vi "Add Noise Single.vi"(6 "Sampling":T2 {"Fs" format="%#_13g"}, 8 "error in (no error)":errorcluster, 10 "Noise Cluster":T1={"1/f vs. Uniform "=0.005, "60Hz Amplitude"=0.005, "Gauss/Unif %"=0.5, "Noise Amp"=0.005}, 11 "signal in":waveform(dbl)) -> (0 "error out":errorcluster, 3 "signal out":waveform(dbl))   [LabVIEW 2019, in "DAQmx.lvclass"]
uses:
  DAQmx.lvclass
  Instrument.DAQ/Typedefs/DAQ.Sampling.Sampling--Cluster.ctl
  <vilib>/measure/NI_MABase.lvlib
  Instrument.DAQ/Instrument.DAQ.lvclass
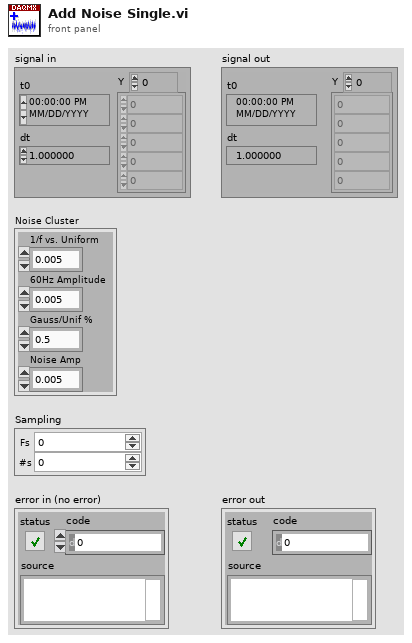
[diagram p1: front panel]
types:
  T1 = cluster{"1/f vs. Uniform ":dbl, "60Hz Amplitude":dbl, "Gauss/Unif %":dbl, "Noise Amp":dbl}
  T2 = typedef "Instrument.Lockin.lvlib/Instrument.DAQ.lvclass/DAQ.Sampling.Sampling--Cluster.ctl" = cluster{"Fs":dbl, "#s":i32}
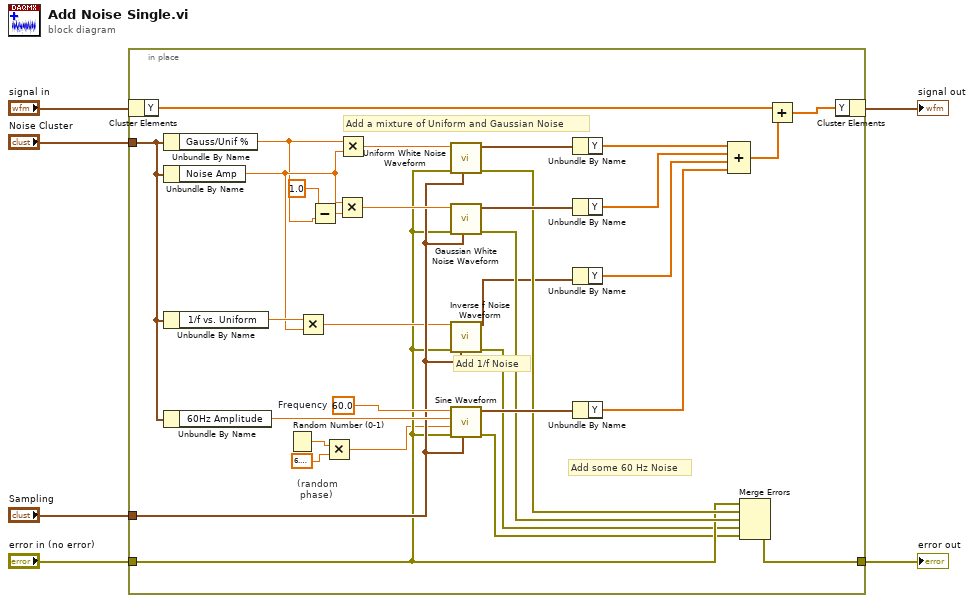
[diagram p0: block diagram]
diagram:
  n1 = in-place {
    in-place-border: "Noise Cluster" -> [w38]
    in-place-border: "Sampling" -> [w21]
    in-place-border: "error in (no error)" -> [w17]
    in-place-border: [w16] -> w4
    w25 = 60.0  # Frequency
    # "(random\n phase)"
    # "Add 1/f Noise"
    # "Add some 60 Hz Noise"
    # "Add a mixture of Uniform and Gaussian Noise"
    n2 = in-place-cluster #1("signal in") -> ("Y"=w14:dbl[])
    n3 = Unbundle By Name(w38) -> ("Gauss/Unif %"=w7:dbl)
    n4 = Unbundle By Name(w38) -> ("Noise Amp"=w22:dbl)
    n5 = Unbundle By Name(w38) -> ("1/f vs. Uniform"=w29:dbl)
    n6 = Unbundle By Name(w38) -> ("60Hz Amplitude"=w28:dbl)
    n7 = Random Number (0-1)() -> (number: 0 to 1=w11:dbl)
    n8 = Multiply(x=w29, y=w22) -> (x*y=w20:dbl)
    n9 = Subtract(x=1.0, y=w7) -> (x-y=w35:dbl)
    n10 = Multiply(x=w11, y=6.283185307179586) -> (x*y=w9:dbl)
    n11 = Multiply(x=w22, y=w35) -> (x*y=w27:dbl)
    n12 = Multiply(x=w7, y=w22) -> (x*y=w26:dbl)
    n13 = call <vilib>:"Uniform White Noise Waveform.vi"("sampling info"=w21, "error in (no error)"=w17, "amplitude"=w26) -> ("error out"=w23:errorcluster, "signal out"=w36:waveform(dbl))  [unwired: 7 in]
    n14 = call <vilib>:"Gaussian White Noise Waveform.vi"("sampling info"=w21, "error in (no error)"=w17, "standard deviation"=w27) -> ("error out"=w24:errorcluster, "signal out"=w37:waveform(dbl))  [unwired: 7 in]
    n15 = call <vilib>:"Inverse f Noise Waveform.vi"("noise density"=w20, "error in (no error)"=w17, "sampling info"=w21) -> ("signal out"=w19:waveform(dbl), "error out"=w12:errorcluster)  [unwired: 8 in, 3 out]
    n16 = call <vilib>:"Sine Waveform.vi"("sampling info"=w21, "error in (no error)"=w17, "phase"=w9, "amplitude"=w28, "frequency"=w25) -> ("error out"=w13:errorcluster, "signal out"=w33:waveform(dbl))  [unwired: 5 in]
    n17 = Unbundle By Name(w36) -> ("Y"=w32:dbl[])
    n18 = Unbundle By Name(w37) -> ("Y"=w30:dbl[])
    n19 = Unbundle By Name(w19) -> ("Y"=w18:dbl[])
    n20 = Unbundle By Name(w33) -> ("Y"=w31:dbl[])
    n21 = Compound Arithmetic op=ADD(w32, w30, w18, w31) -> (w15:dbl[])
    n22 = Merge Errors(w17, w23, w24, w12, w13) -> (w16:errorcluster)
    n23 = Add(x=w14, y=w15) -> (x+y=w8:dbl[])
    n24 = in-place-cluster #1("Y"=w8) -> (→"signal out":waveform(dbl))
  }
  "error out" <- w4
